vi "FRC-Traj-Lib-analog-pid-complex-test.vi"() -> ()   [LabVIEW 2019]
uses:
  <vilib>/Rock Robotics/WPI/ThirdParty/JAS_Junk/TrajLib/PID_CONTROLLER.ctl
  <vilib>/Rock Robotics/WPI/ThirdParty/JAS_Junk/TrajLib/LinearFilter_ResetToValue.vi
  <vilib>/Rock Robotics/WPI/ThirdParty/JAS_Junk/TrajLib/LinearFilter_Calculate.vi
  <vilib>/Rock Robotics/WPI/ThirdParty/JAS_Junk/TrajLib/PIDController_Calculate_SP_PV.vi
  <vilib>/Rock Robotics/WPI/ThirdParty/JAS_Junk/TrajLib/PIDController_AtSetpoint.vi
  <vilib>/Rock Robotics/WPI/ThirdParty/JAS_Junk/TrajLib/PIDController_SetPID.vi
  <vilib>/Rock Robotics/WPI/ThirdParty/JAS_Junk/TrajLib/PIDController_SetIntegratorRange.vi
  <vilib>/Rock Robotics/WPI/ThirdParty/JAS_Junk/TrajLib/PIDController_SetTolerancePandV.vi
  <vilib>/Rock Robotics/WPI/ThirdParty/JAS_Junk/TrajLib/PIDController_DisableContinousInput.vi
  <vilib>/Rock Robotics/WPI/ThirdParty/JAS_Junk/TrajLib/PIDController_EnableContinousInput.vi
  <vilib>/Rock Robotics/WPI/ThirdParty/JAS_Junk/TrajLib/PIDController_Reset.vi
  <vilib>/Rock Robotics/WPI/ThirdParty/JAS_Junk/TrajLib/PIDController_NewPeriod.vi
  <vilib>/Rock Robotics/WPI/ThirdParty/JAS_Junk/TrajLib/PIDController_SetSetpoint.vi
  <vilib>/Rock Robotics/WPI/ThirdParty/JAS_Junk/TrajLib/PIDController_Calculate_PV.vi
  <vilib>/Rock Robotics/WPI/ThirdParty/JAS_Junk/TrajLib/ControllerUtil_GetModulusError.vi
  <vilib>/Rock Robotics/SystemInterfaces/NetworkCommunication/NetComm_UsageReport_report.vi
  <vilib>/Rock Robotics/WPI/ThirdParty/JAS_Junk/TrajLib/Util_LibraryGlobals.vi
  <vilib>/addons/control/pid/pid.llb/PID Lead-Lag (DBL).vi
  <vilib>/Rock Robotics/WPI/ThirdParty/JAS_Junk/TrajLib/LinearFilter_MovingAverage.vi
  <vilib>/Rock Robotics/WPI/ThirdParty/JAS_Junk/TrajLib/LinearFilter_LowPassBW1.vi
  <vilib>/Rock Robotics/WPI/ThirdParty/JAS_Junk/TrajLib/LinearFilter_LowPassBW2.vi
  <vilib>/Rock Robotics/WPI/ThirdParty/JAS_Junk/TrajLib/LinearFilter_HighPassBW1.vi
  <vilib>/Rock Robotics/WPI/ThirdParty/JAS_Junk/TrajLib/LinearFilter_HighPassBW2.vi
  <vilib>/addons/control/pid/NI_PID_pid.lvlib
  <vilib>/Rock Robotics/WPI/ThirdParty/JAS_Junk/TrajLib/Trajectory_Library.lvlib
panel:
  in  "Tab Control":T1(tab)
  in  "Enable Noise":bool=TRUE
  in  "Auto / Manual":bool=TRUE
  out "Dash Speed Demand":dbl format="%10.2f"
  in  "Desired Speed":dbl(slide)=-0.22222222222222499 scale=-50.0..50.0 scale format="%#.1f"
  out "Dash Speed Target":dbl format="%10.2f"
  out "DashRightMotorOutput":dbl format="%11.3f"
  out "DashRight Wheel Speed":dbl(knob)=-2.895988890827539e-05 scale=-60.0..60.0
  out "Right Wheel ErrorFilt":dbl format="%11.3f"
  out "Right Wheel SpeedFilt":dbl format="%10.2f"
  out "DashLeft Wheel Speed":dbl(knob)=-2.895988890827539e-05 scale=-60.0..60.0
  out "Left Wheel ErrorFilt":dbl format="%11.3f"
  out "DashLeftMotorOutput":dbl format="%11.3f"
  out "Left Wheel Speed Filt":dbl format="%10.2f"
  out "Left CO":dbl format="%13.3f"
  out "Right CO":dbl format="%13.3f"
  out "Duration":dbl format="%11.3f"
  out "Late":dbl format="%11.3f"
  out "SP, PV, CO Left":T2(graph)
  out "SP, PV, CO Right":T2(graph)
  in  "SetPoint Change Rate":dbl=80.0 min=1.0 max=9000.0 format="%14.4f"
  in  "PID Tuning Left":T3={"Kp"=0.4, "Ki"=2.0, "Kd"=0.0, "MaximumIntegral"=1.5, "MinimumIntegral"=-1.5}
  in  "PID Tuning Right":T3={"Kp"=0.4, "Ki"=2.0, "Kd"=0.0, "MaximumIntegral"=1.5, "MinimumIntegral"=-1.5}
  out "Left PID Data":T4={"Kp"=0.0, "Ki"=0.0, "Kd"=0.0, "Period"=0.0, "Max_Integral"=0.0, "Min_Integral"=0.0, "Max_Input"=0.0, "Min_Input"=0.0, "Continuous"=FALSE, "PositionError"=0.0, "VelocityError"=0.0, "PrevError"=0.0, "TotalError"=0.0, "PositionTolerance"=0.0, "VelocityTolerance"=0.0, "SetPoint"=0.0, "Kf"=0.0, "Prev_Deriv"=0.0, "Prev_Deriv 2"=0.0, "DerivativeFilter"=FALSE, "Min_Output"=-9.99e+35, "Max_Output"=9.9e+35, "Prev_F_P"=0.0, "Prev_F_P_2"=0.0, "AntiWindupActive"=FALSE, "Measurement"=0.0} {"Measurement" format="%16_6e"; "Prev_F_P_2" format="%16_6e"; "Prev_F_P" format="%16_6e"; "Max_Output" format="%16_6e"; "Min_Output" format="%16_6e"; "Prev_Deriv 2" format="%16_6e"; "Prev_Deriv" format="%16_6e"; "Kf" format="%16_6e"; "SetPoint" format="%16_6e"; "VelocityTolerance" format="%16_6e"; "PositionTolerance" format="%16_6e"; "TotalError" format="%16_6e"; "PrevError" format="%16_6e"; "VelocityError" format="%16_6e"; "PositionError" format="%16_6e"; "Min_Input" format="%16_6e"; "Max_Input" format="%16_6e"; "Min_Integral" format="%16_6e"; "Max_Integral" format="%16_6e"; "Period" format="%16_6e"; "Kd" format="%16_6e"; "Ki" format="%16_6e"; "Kp" format="%16_6e"}
  out "Right PID Data":T4={"Kp"=0.0, "Ki"=0.0, "Kd"=0.0, "Period"=0.0, "Max_Integral"=0.0, "Min_Integral"=0.0, "Max_Input"=0.0, "Min_Input"=0.0, "Continuous"=FALSE, "PositionError"=0.0, "VelocityError"=0.0, "PrevError"=0.0, "TotalError"=0.0, "PositionTolerance"=0.0, "VelocityTolerance"=0.0, "SetPoint"=0.0, "Kf"=0.0, "Prev_Deriv"=0.0, "Prev_Deriv 2"=0.0, "DerivativeFilter"=FALSE, "Min_Output"=-9.99e+35, "Max_Output"=9.9e+35, "Prev_F_P"=0.0, "Prev_F_P_2"=0.0, "AntiWindupActive"=FALSE, "Measurement"=0.0} {"Measurement" format="%16_6e"; "Prev_F_P_2" format="%16_6e"; "Prev_F_P" format="%16_6e"; "Max_Output" format="%16_6e"; "Min_Output" format="%16_6e"; "Prev_Deriv 2" format="%16_6e"; "Prev_Deriv" format="%16_6e"; "Kf" format="%16_6e"; "SetPoint" format="%16_6e"; "VelocityTolerance" format="%16_6e"; "PositionTolerance" format="%16_6e"; "TotalError" format="%16_6e"; "PrevError" format="%16_6e"; "VelocityError" format="%16_6e"; "PositionError" format="%16_6e"; "Min_Input" format="%16_6e"; "Max_Input" format="%16_6e"; "Min_Integral" format="%16_6e"; "Max_Integral" format="%16_6e"; "Period" format="%16_6e"; "Kd" format="%16_6e"; "Ki" format="%16_6e"; "Kp" format="%16_6e"}
  in  "RightWheelNoise":dbl
  in  "LeftWheelNoise":dbl
  out "RightWheelSpeed":dbl
  out "LeftWheelSpeed":dbl
  out "RightMotorOutput":dbl
  out "LeftMotorOutput":dbl
  out "SpeedSetpoint":dbl
  in  "SpeedTarget":dbl
  in  "SpeedControlEnabled":bool
  # "Example of Closed Loop Motor Speed Control\n(Simple Example 003)"
  # "Enter a desired speed and then press the Set Speed Target \nbutton.  This simulates the joystick input."
  # "This value shows the current speed of each wheel.  This is measured by an encoder.  The encoder measures\n speed by counting pulses of the wheel turning and dividing by the time interval.  Total distance change\nis also a result.  This value is called the \"Process Variable\"."
  # "FT/SEC"
  # "FT/SEC"
  # "FT/SEC"
  # "FT/SEC"
  # "The Speed Target is rate limited so not to make\nto drastic a change in the desired speed.  (This is\nwhat happens mechanically when pushing the gas\npedal of a real car.)"
  # "This error value shows the error between the current speed\nand the speed demand."
  # "FT/SEC"
  # "This example adds a \"Manual\" mode so that the still operates\nif the encoder fails."
  # "FT/SEC"
  # "FT/SEC"
  # "This value shows the current motor output demand.  This could also be a motor speed demand and \nanother closed loop controller would control the motor speed.  In this simple example this value is \nused to drive the simulated motor directly.  This motor demand is called the \"Control Output\"."
  # "Enables some simulated process noise"
  # "FT/SEC/SEC"
  # "These are the tuning parameters for the PID VI"
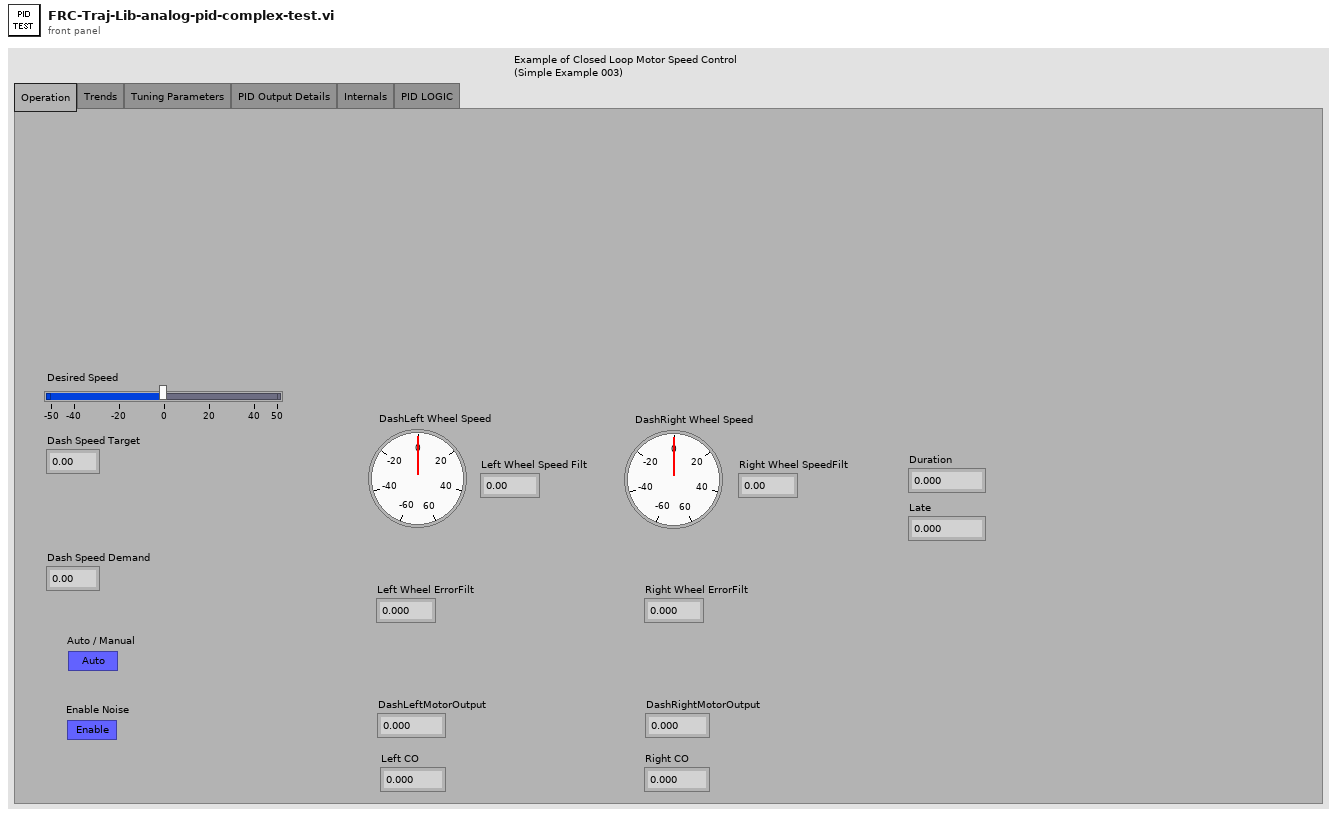
[diagram p1: front panel]
types:
  T1 = enum32{"Operation", "Trends", "Tuning Parameters", "PID Output Details", "Internals", "PID LOGIC"}
  T2 = cluster{"MotorDemand":dbl, "CurrentSetpoint":dbl, "CurrentPosition":dbl}
  T3 = cluster{"Kp":dbl, "Ki":dbl, "Kd":dbl, "MaximumIntegral":dbl, "MinimumIntegral":dbl}
  T4 = typedef "Trajectory_Library.lvlib/PID_CONTROLLER.ctl" = cluster{"Kp":dbl, "Ki":dbl, "Kd":dbl, "Period":dbl, "Max_Integral":dbl, "Min_Integral":dbl, "Max_Input":dbl, "Min_Input":dbl, "Continuous":bool, "PositionError":dbl, "VelocityError":dbl, "PrevError":dbl, "TotalError":dbl, "PositionTolerance":dbl, "VelocityTolerance":dbl, "SetPoint":dbl, "Kf":dbl, "Prev_Deriv":dbl, "Prev_Deriv 2":dbl, "DerivativeFilter":bool, "Min_Output":dbl, "Max_Output":dbl, "Prev_F_P":dbl, "Prev_F_P_2":dbl, "AntiWindupActive":bool, "Measurement":dbl}
  T5 = cluster{"gain":dbl, "lag time":dbl, "lead time":dbl}
  T6 = enum16{"Moving Average", "Low Pass 1st Order Butterworth", "Low Pass 2nd Order Butterworth", "High Pass 1st Order Butterworth", "High Pass 2nd Order Butterworth"}
  T7 = cluster{"LeftMotorOutput":dbl, "SpeedSetpoint":dbl, "LeftWheelSpeed":dbl}
  T8 = cluster{"RightMotorOutput":dbl, "SpeedSetpoint":dbl, "RightWheelSpeed":dbl}
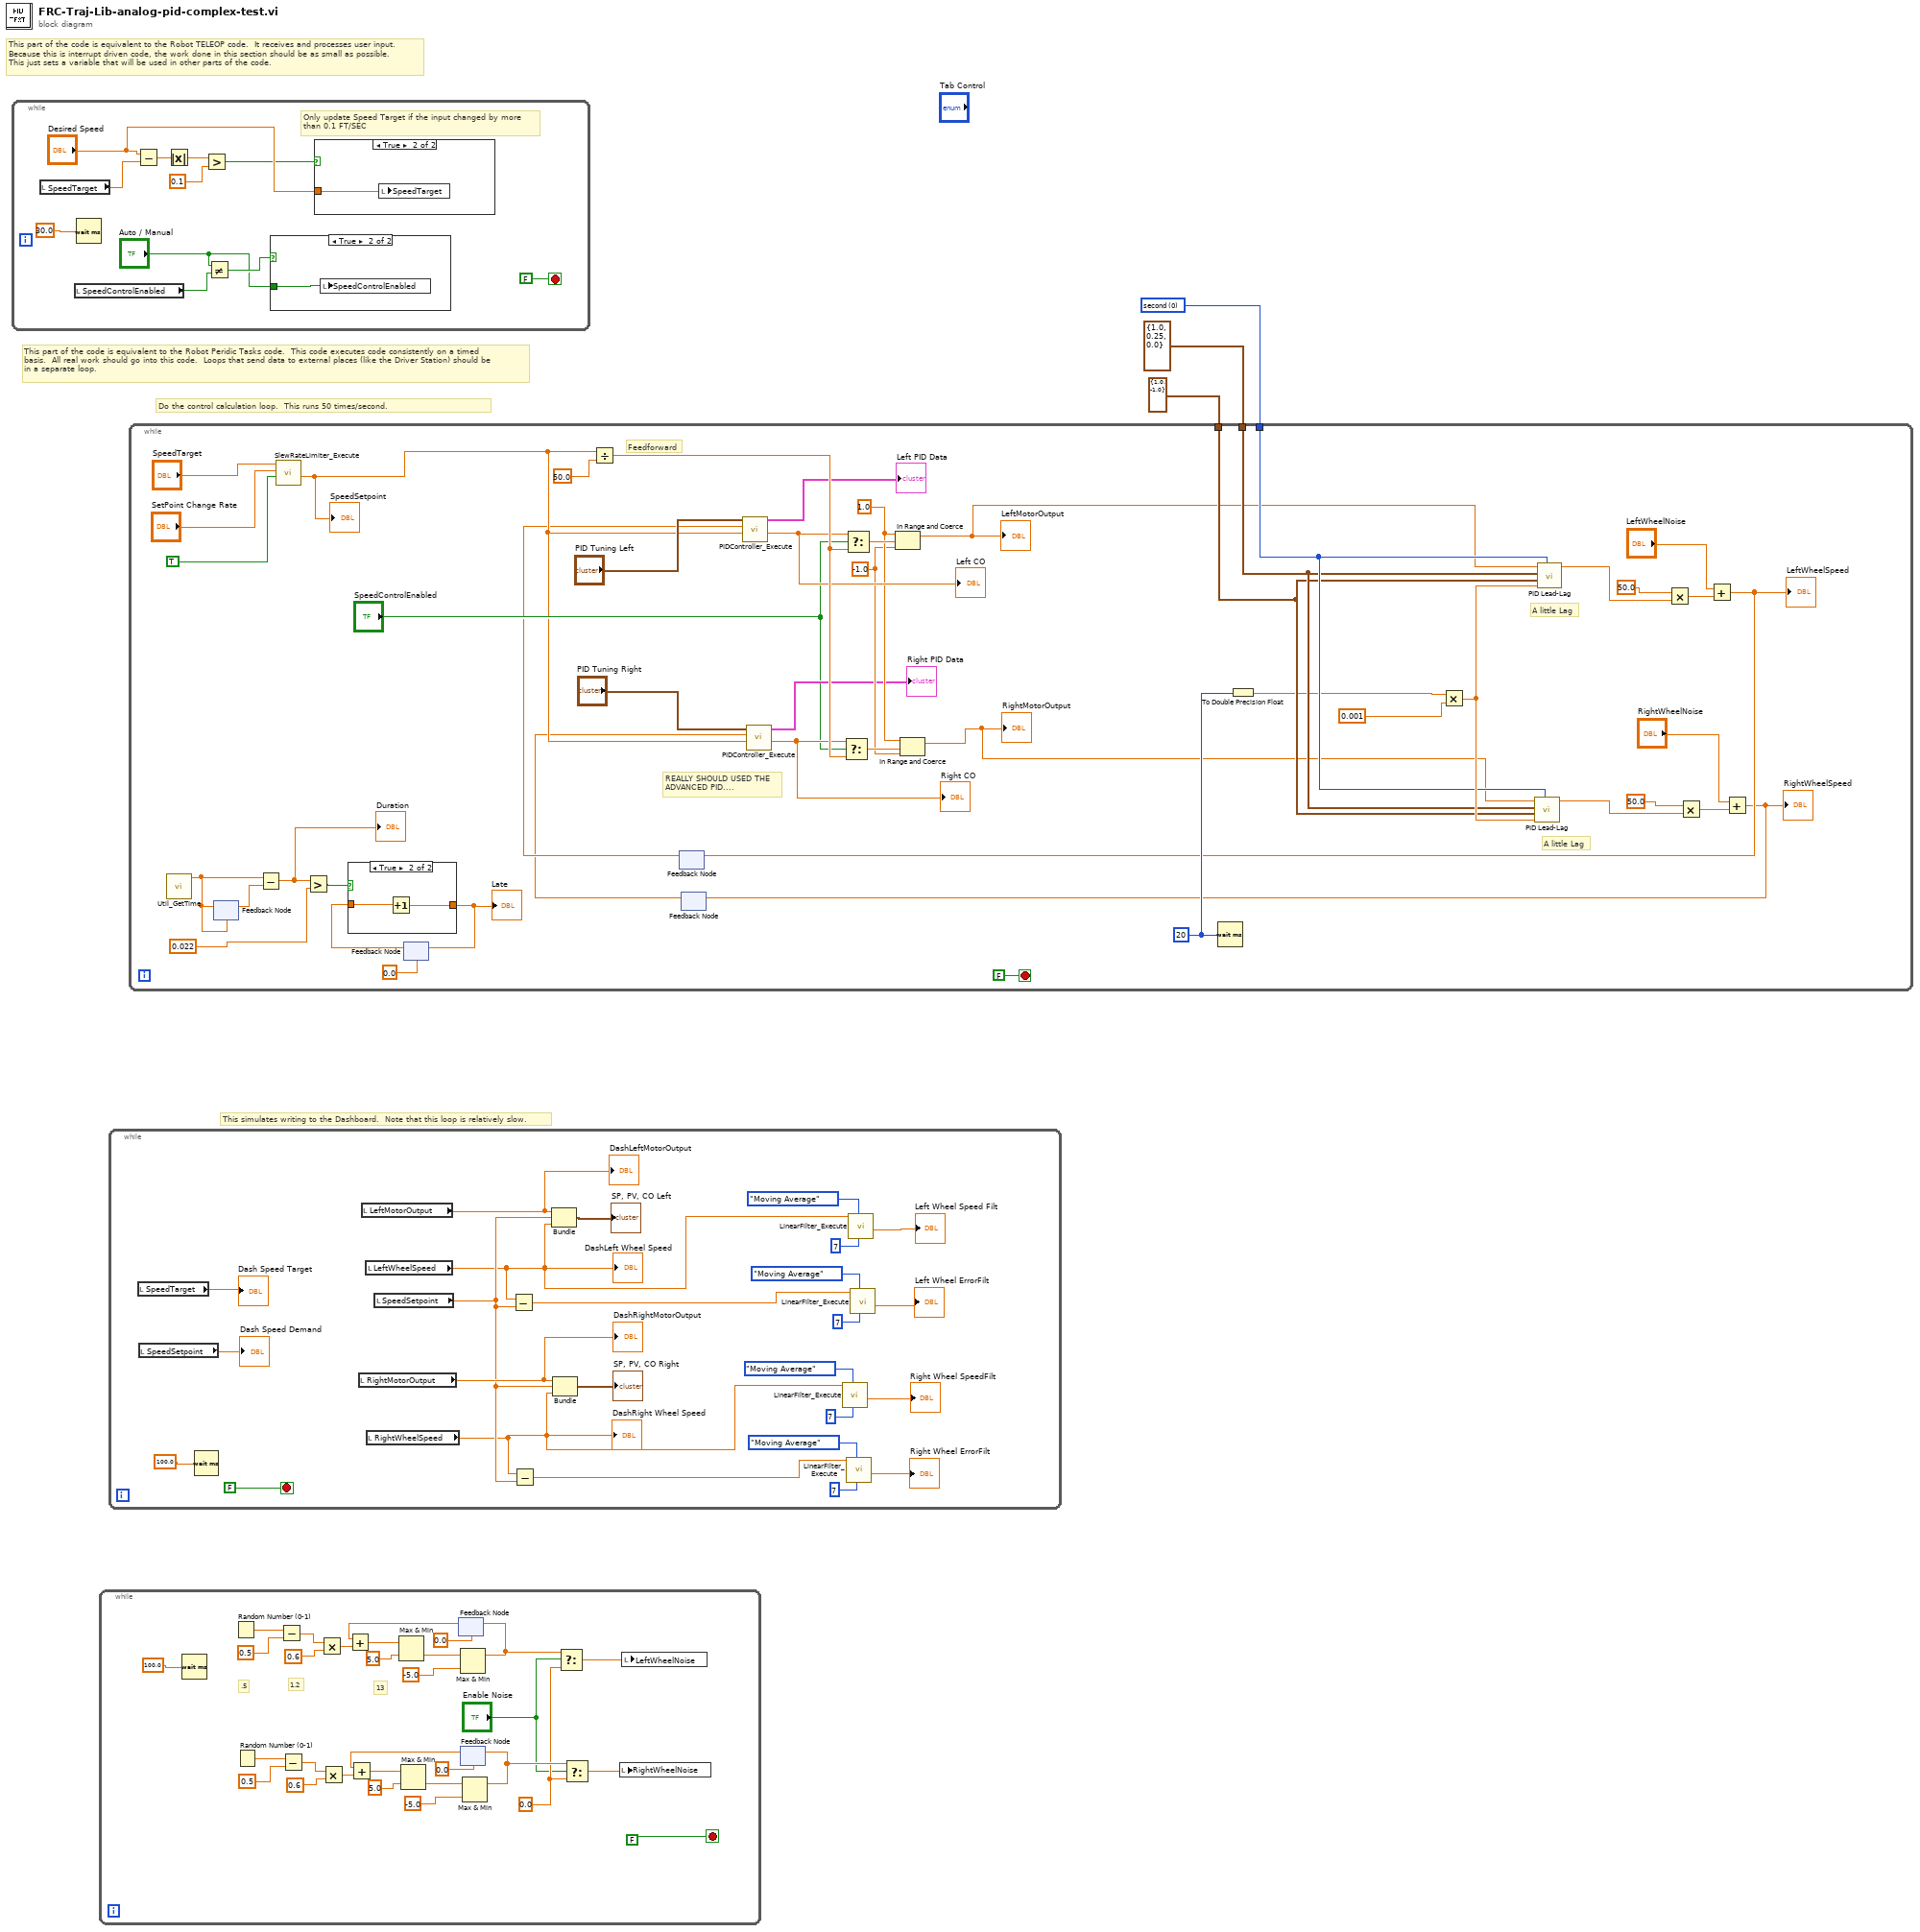
[diagram p0: block diagram]
diagram:
  w3 = u16 0 items=["second", "minute"] ("time unit")
  # "This simulates writing to the Dashboard.  Note that this loop is relatively slow."
  # "Do the control calculation loop.  This runs 50 times/second."
  # "This part of the code is equivalent to the Robot Peridic Tasks code.  This code executes code consistently on a timed\nbasis.  All real work should go into this code.  Loops that send data to external places (like the Driver Station) should be \nin a separate loop."
  # "This part of the code is equivalent to the Robot TELEOP code.  It receives and processes user input.\nBecause this is interrupt driven code, the work done in this section should be as small as possible.\nThis just sets a variable that will be used in other parts of the code."
  n1 = while {
    stop <- FALSE stop-if-true
    # "Only update Speed Target if the input changed by more\nthan 0.1 FT/SEC"
    n2 = local read "SpeedTarget"() -> (w13:dbl)
    n3 = local read "SpeedControlEnabled"() -> (w5:bool)
    n4 = Wait (ms)(milliseconds to wait=30.0) -> ()  [unwired: 1 out]
    n5 = Subtract(x="Desired Speed", y=w13) -> (x-y=w12:dbl)
    n6 = Absolute Value(x=w12) -> (abs(x)=w11:dbl)
    n7 = Greater?(x=w11, y=0.1) -> (0:w8:bool)
    n8 = Not Equal?(x="Auto / Manual", y=w5) -> (x != y?=w6:bool)
    n9 = case shown="True" w6 {
      tunnel: "Auto / Manual" -> [_ w15]
      frame False {
      }
      frame True {
        n10 = local write "SpeedControlEnabled"(w15) -> ()
      }
    }
    n11 = case shown="True" w8 {
      tunnel: "Desired Speed" -> [_ w16]
      frame False {
      }
      frame True {
        n12 = local write "SpeedTarget"(w16) -> ()
      }
    }
  }
  n13 = while {
    stop <- FALSE stop-if-true
    w20 = 0.0 ("f")
    # "13"
    # "1.2"
    # ".5"
    n14 = Wait (ms)(milliseconds to wait=100.0) -> ()  [unwired: 1 out]
    n15 = Random Number (0-1)() -> (number: 0 to 1=w18:dbl)
    n16 = Random Number (0-1)() -> (number: 0 to 1=w17:dbl)
    n17 = Subtract(x=w18, y=0.5) -> (x-y=w37:dbl)
    n18 = Subtract(x=w17, y=0.5) -> (x-y=w27:dbl)
    n19 = Multiply(x=w37, y=0.6) -> (x*y=w36:dbl)
    n20 = Multiply(x=w27, y=0.6) -> (x*y=w26:dbl)
    n21 = feedback #1(0.0) -> (w39:dbl)
    n22 = Add(x=w39, y=w36) -> (x+y=w43:dbl)
    n23 = Max & Min(x=w43, y=5.0) -> (min(x,y)=w42:dbl)  [unwired: 1 out]
    n24 = Max & Min(x=w42, y=-5.0) -> (max(x,y)=w23:dbl)  [unwired: 1 out]
    n25 = feedback-in #1(w23) -> ()
    n26 = feedback #2(0.0) -> (w29:dbl)
    n27 = Add(x=w29, y=w26) -> (x+y=w33:dbl)
    n28 = Max & Min(x=w33, y=5.0) -> (min(x,y)=w32:dbl)  [unwired: 1 out]
    n29 = Max & Min(x=w32, y=-5.0) -> (max(x,y)=w21:dbl)  [unwired: 1 out]
    n30 = feedback-in #2(w21) -> ()
    n31 = Select(t=w23, s="Enable Noise", f=w20) -> (s? t:f=w24:dbl)
    n32 = Select(t=w21, s="Enable Noise", f=w20) -> (s? t:f=w22:dbl)
    n33 = local write "RightWheelNoise"(w22) -> ()
    n34 = local write "LeftWheelNoise"(w24) -> ()
  }
  n35 = while {
    stop <- FALSE stop-if-true
    n36 = local read "SpeedTarget"() -> (→"Dash Speed Target":dbl)
    n37 = local read "SpeedSetpoint"() -> (→"Dash Speed Demand":dbl)
    n38 = Wait (ms)(milliseconds to wait=100.0) -> ()  [unwired: 1 out]
    n39 = local read "RightMotorOutput"() -> (w67:dbl)
    "DashRightMotorOutput" <- w67
    n40 = local read "LeftMotorOutput"() -> (w64:dbl)
    "DashLeftMotorOutput" <- w64
    n41 = local read "LeftWheelSpeed"() -> (w60:dbl)
    "DashLeft Wheel Speed" <- w60
    n42 = local read "RightWheelSpeed"() -> (w51:dbl)
    "DashRight Wheel Speed" <- w51
    n43 = local read "SpeedSetpoint"() -> (w63:dbl)
    n44 = Subtract(x=w60, y=w63) -> (x-y=w56:dbl)
    n45 = Subtract(x=w51, y=w63) -> (x-y=w47:dbl)
    n46 = Bundle("LeftMotorOutput"=w64, "SpeedSetpoint"=w63, "LeftWheelSpeed"=w60) -> (→"SP, PV, CO Left":T7)  [unwired: 1 in]
    n47 = Bundle("RightMotorOutput"=w67, "SpeedSetpoint"=w63, "RightWheelSpeed"=w51) -> (→"SP, PV, CO Right":T8)  [unwired: 1 in]
    n48 = call <vilib>:"LinearFilter_Execute.vi"("Samples"=7, "Filter Type"=T6."Moving Average", "Input"=w51) -> ("Output"=→"Right Wheel SpeedFilt":dbl)  [unwired: 7 in, 1 out]
    n49 = call <vilib>:"LinearFilter_Execute.vi"("Samples"=7, "Filter Type"=T6."Moving Average", "Input"=w47) -> ("Output"=→"Right Wheel ErrorFilt":dbl)  [unwired: 7 in, 1 out]
    n50 = call <vilib>:"LinearFilter_Execute.vi"("Samples"=7, "Filter Type"=T6."Moving Average", "Input"=w60) -> ("Output"=→"Left Wheel Speed Filt":dbl)  [unwired: 7 in, 1 out]
    n51 = call <vilib>:"LinearFilter_Execute.vi"("Samples"=7, "Filter Type"=T6."Moving Average", "Input"=w56) -> ("Output"=→"Left Wheel ErrorFilt":dbl)  [unwired: 7 in, 1 out]
  }
  n52 = while {
    tunnel: w3 -> [w83]
    tunnel: T5 {"gain"=1.0, "lag time"=0.25, "lead time"=0.0} ("tuning parameters") -> [w82]
    tunnel: cluster{"output high":dbl, "output low":dbl} {"output high"=1.0, "output low"=-1.0} ("output range") -> [w81]
    stop <- FALSE stop-if-true
    w107 = -1.0 ("lower limit")
    w108 = 1.0 ("upper limit")
    w80 = u32 20 ("milliseconds to wait")
    # "A little Lag"
    # "A little Lag"
    # "REALLY SHOULD USED THE\nADVANCED PID...."
    # "Feedforward"
    n53 = call <vilib>:"Util_GetTime.vi"() -> ("FPGA_Time_Seconds"=w101:dbl)  [unwired: 10 in, 1 out]
    n54 = feedback #3(w101) -> (w100:dbl)
    n55 = feedback-in #3(w101) -> ()
    n56 = Subtract(x=w101, y=w100) -> (x-y=w98:dbl)
    "Duration" <- w98
    n57 = call <vilib>:"SlewRateLimiter_Execute.vi"("Enable"=TRUE, "Rate"="SetPoint Change Rate", "Input"="SpeedTarget") -> ("Output"=w93:dbl)  [unwired: 7 in, 1 out]
    "SpeedSetpoint" <- w93
    n58 = Greater?(x=w98, y=0.022) -> (0:w99:bool)
    n59 = feedback #4(0.0) -> (w102:dbl)
    n60 = case shown="True" w99 {
      tunnel: [w119 w121] -> w103
      tunnel: w102 -> [w119 w120]
      frame False {
      }
      frame True {
        n61 = Increment(x=w120) -> (x+1=w121:dbl)
      }
    }
    "Late" <- w103
    n62 = feedback-in #4(w103) -> ()
    n63 = Divide(x=w93, y=50.0) -> (x/y=w117:dbl)
    n64 = feedback #5() -> (w74:dbl)  [unwired: 1 in]
    n65 = feedback #6() -> (w73:dbl)  [unwired: 1 in]
    n66 = call <vilib>:"PIDController_Execute.vi"("SP-SetPoint"=w93, "PV-Measurement"=w74, "PID Tuning"="PID Tuning Left") -> ("CO-ControlOutput"=w111:dbl, "out PID_CONTROLLER"=→"Left PID Data":T4)  [unwired: 6 in, 1 out]
    "Left CO" <- w111
    n67 = call <vilib>:"PIDController_Execute.vi"("SP-SetPoint"=w93, "PV-Measurement"=w73, "PID Tuning"="PID Tuning Right") -> ("CO-ControlOutput"=w104:dbl, "out PID_CONTROLLER"=→"Right PID Data":T4)  [unwired: 6 in, 1 out]
    "Right CO" <- w104
    n68 = Select(t=w104, s="SpeedControlEnabled", f=w117) -> (s? t:f=w109:dbl)
    n69 = Select(t=w111, s="SpeedControlEnabled", f=w117) -> (s? t:f=w110:dbl)
    n70 = In Range and Coerce(upper limit=w108, x=w110, lower limit=w107) -> (coerced(x)=w78:dbl)  [unwired: 1 out]
    "LeftMotorOutput" <- w78
    n71 = In Range and Coerce(upper limit=w108, x=w109, lower limit=w107) -> (coerced(x)=w77:dbl)  [unwired: 1 out]
    "RightMotorOutput" <- w77
    n72 = Wait (ms)(milliseconds to wait=w80) -> ()  [unwired: 1 out]
    n73 = To Double Precision Float(number=w80) -> (double precision float=w79:dbl)
    n74 = Multiply(x=w79, y=0.001) -> (x*y=w91:dbl)
    n75 = call-poly <vilib>:"PID Lead-Lag.vi"("time unit"=w83, "dt (s)"=w91, "output range"=w81, "tuning parameters"=w82, "input"=w77) -> ("output"=w72:dbl)  [unwired: 3 in, 1 out]
    n76 = call-poly <vilib>:"PID Lead-Lag.vi"("time unit"=w83, "dt (s)"=w91, "output range"=w81, "tuning parameters"=w82, "input"=w78) -> ("output"=w92:dbl)  [unwired: 3 in, 1 out]
    n77 = Multiply(x=50.0, y=w92) -> (x*y=w88:dbl)
    n78 = Multiply(x=50.0, y=w72) -> (x*y=w87:dbl)
    n79 = Add(x="LeftWheelNoise", y=w88) -> (x+y=w76:dbl)
    "LeftWheelSpeed" <- w76
    n80 = feedback-in #5(w76) -> ()
    n81 = Add(x="RightWheelNoise", y=w87) -> (x+y=w75:dbl)
    "RightWheelSpeed" <- w75
    n82 = feedback-in #6(w75) -> ()
  }
